vi "CMI ADS127L21 - Select Channels.vi"(8 "error in (no error)":errorcluster, 10 "Channels List ([1,2])":i32[](array[numeric])=[1, 2] min=1 max=8 step=1, 11 "session in":T1 {"channels"."Channel" min=1 max=8 step=1; "channels"."Range [Vpk]" items=["±1.65V", "±2V"]}) -> (0 "error out":errorcluster, 3 "session out":T1 {"channels"."Channel" min=1 max=8 step=1; "channels"."Range [Vpk]" items=["±1.65V", "±2V"]})   [LabVIEW 2020]
doc: "Sets channels list for recording."
uses:
  CMI ADS127L21 - Session.ctl
  CMI ADS127L21 - Record Channel.ctl
  CMI ADS127L21 - Input Range.ctl
  CMI ADS127L21 - Input Mode.ctl
  CMI ADS127L21 - Input Impedance.ctl
  CMI ADS127L21 - EXTOUT Mode.ctl
  CMI ADS127L21 - EXTOUT Polarity.ctl
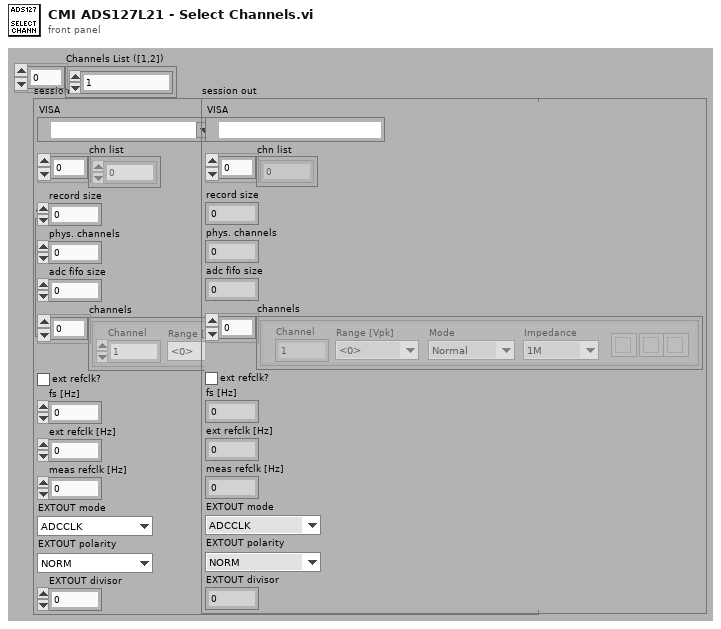
[diagram p1: front panel]
types:
  T1 = typedef "CMI ADS127L21 - Session.ctl" = cluster{"VISA":refnum<visa-resource-name>, "chn list":i32[], "record size":i32, "phys. channels":i32, "adc fifo size":i32, "channels":T2[], "ext refclk?":bool, "fs [Hz]":dbl, "ext refclk [Hz]":dbl, "meas refclk [Hz]":dbl, "EXTOUT mode":T6, "EXTOUT polarity":T7, "EXTOUT divisor":i32}
  T2 = typedef "CMI ADS127L21 - Record Channel.ctl" = cluster{"Range [Vpk]":T3, "Channel":i32, "Mode":T4, "Impedance":T5, "btn clr":bool, "btn up":bool, "btn down":bool}
  T3 = typedef "CMI ADS127L21 - Input Range.ctl" = dbl
  T4 = typedef "CMI ADS127L21 - Input Mode.ctl" = enum16{"Normal", "Inverted", "GND"}
  T5 = typedef "CMI ADS127L21 - Input Impedance.ctl" = enum16{"1M", "1k5"}
  T6 = typedef "CMI ADS127L21 - EXTOUT Mode.ctl" = enum16{"ADCCLK", "REFCLK", "SMPLCLK", "FIRST"}
  T7 = typedef "CMI ADS127L21 - EXTOUT Polarity.ctl" = enum16{"NORM", "INV"}
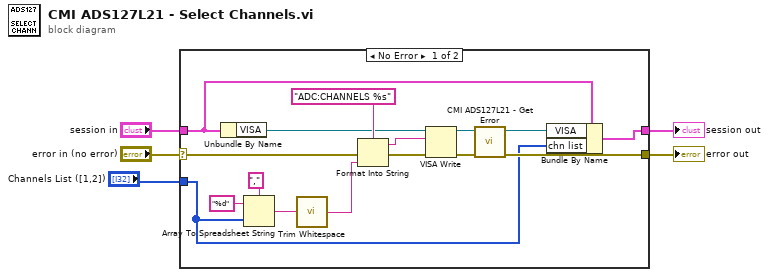
[diagram p0: block diagram]
diagram:
  n1 = case shown="No Error" "error in (no error)" {
    selector: "error in (no error)" -> [w16 w23]
    tunnel: "session in" -> [w7 w22]
    tunnel: [w8 w22] -> w4
    tunnel: [w18 w23] -> w3
    tunnel: "Channels List ([1,2])" -> [w6 _]
    frame No Error {
      n2 = Unbundle By Name(w7) -> ("VISA"=w9:refnum<visa-resource-name>)
      n3 = Array To Spreadsheet String(delimiter (Tab)=",", array=w6, 3:"%d" ("format string")) -> (spreadsheet string=w11:string)
      n4 = call <vilib>:"Trim Whitespace.vi"("string"=w11) -> ("trimmed string"=w10:string)  [unwired: 1 in]
      n5 = Format Into String(format string="ADC:CHANNELS %s", error in=w16, w10) -> (resulting string=w14:string, error out=w15:errorcluster)  [unwired: 1 in]
      n6 = VISA Write(VISA resource name=w9, write buffer=w14, error in (no error)=w15) -> (VISA resource name out=w20:refnum<visa-resource-name>, error out=w21:errorcluster)  [unwired: 1 out]
      n7 = call "CMI ADS127L21 - Get Error.vi"("error in (no error)"=w21, "VISA in"=w20) -> ("error out"=w18:errorcluster, "VISA out"=w19:refnum<visa-resource-name>)  [unwired: 8 in]
      n8 = Bundle By Name(cluster=w7, "VISA"=w19, "chn list"=w6) -> (w8:T1)
    }
    frame Error {
    }
  }
  "error out" <- w3
  "session out" <- w4
